vi "oa_TV Pulse Position (1Chan).vi"(4 "slope (Rising)":u16(ring) items=["Rising", "Falling"], 5 "reset? (F)":bool, 6 "pulse width (2)":i32=2, 7 "missing pulses? (no:F)":bool, 8 "error in (no error)":errorcluster, 9 "hysteresis(0)":dbl format="%.2f", 10 "threshold (auto)":dbl=inf format="%.2f", 11 "analog tacho signal":waveform(dbl)={"t0"=timestamp(0 s since 1904-01-01), "dt"=0.0, "Y"=[]}) -> (0 "error out":errorcluster, 2 "duration":dbl, 3 "pulse positions [s]":dbl[](array[numeric]))   [LabVIEW 2017, in "SoundVib_Torsional.lvlib"]
uses:
  <vilib>/addons/Sound and Vibration/Order Analysis/Torsional Vibration/SoundVib_Torsional.lvlib
  <vilib>/addons/Sound and Vibration/Order Analysis/Tach Process/SubVIs/OAT Edge Detection (1 Tach).vi
  <vilib>/addons/Sound and Vibration/Order Analysis/Tach Process/SoundVib_TachProcess.lvlib
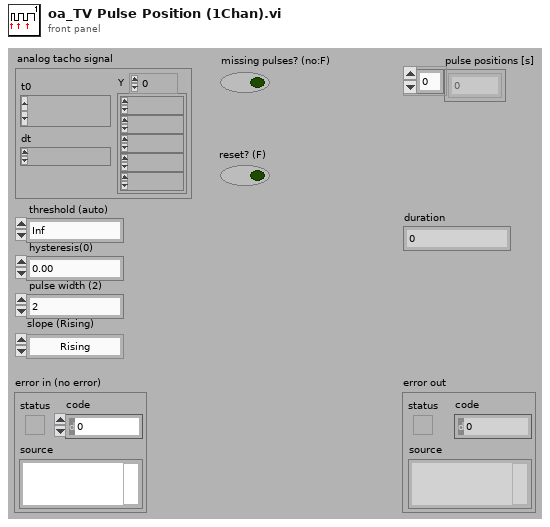
[diagram p1: front panel]
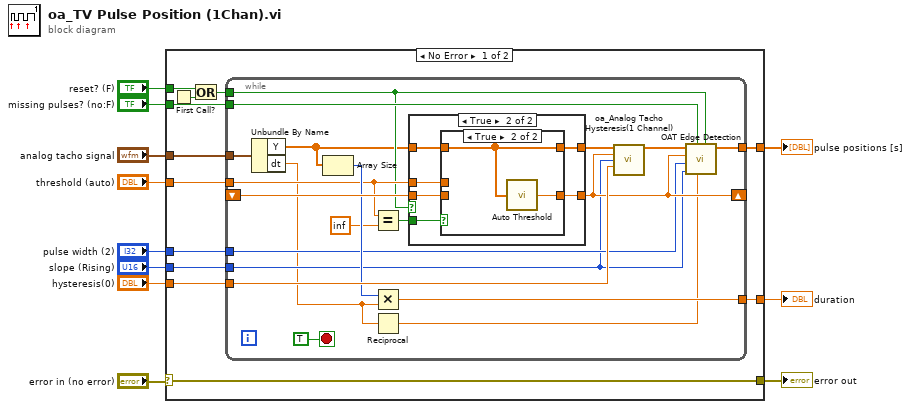
[diagram p0: block diagram]
diagram:
  n1 = case shown="No Error" "error in (no error)" {
    selector: "error in (no error)" -> [w21 w56]
    tunnel: "analog tacho signal" -> [w12 _]
    tunnel: [w21 w56] -> w10
    tunnel: "threshold (auto)" -> [w20 _]
    tunnel: [w14 _] -> w1
    tunnel: [w16 _] -> w7
    tunnel: "reset? (F)" -> [w22 _]
    tunnel: "missing pulses? (no:F)" -> [w15 _]
    tunnel: "hysteresis(0)" -> [w18 _]
    tunnel: "slope (Rising)" -> [w19 _]
    tunnel: "pulse width (2)" -> [w13 _]
    frame No Error {
      n2 = First Call?() -> (First Call?: T/F=w23:bool)
      n3 = Or(x=w22, y=w23) -> (x .or. y?=w17:bool)
      n4 = while {
        shift-right: [w33] -> _
        shift-left: _ -> [w43]
        tunnel: w17 -> [w29]
        tunnel: w20 -> [w36]
        tunnel: w19 -> [w31]
        tunnel: w18 -> [w40]
        tunnel: [w38] -> w16
        tunnel: w15 -> [w34]
        tunnel: w13 -> [w32]
        tunnel: [w27] -> w14
        tunnel: w12 -> [w24]
        stop <- TRUE stop-if-true
        n5 = Unbundle By Name(w24) -> ("Y"=w26:dbl[], "dt"=w25:dbl)
        n6 = Array Size(array=w26) -> (size(s)=w39:i32)
        n7 = Equal?(x=w36, y=inf) -> (x = y?=w35:bool)
        n8 = Multiply(x=w39, y=w25) -> (x*y=w38:dbl)
        n9 = Reciprocal(x=w25) -> (1/x=w30:dbl)
        n10 = case shown="True" w29 {
          tunnel: w26 -> [w44 w51]
          tunnel: [w45 w50] -> w33
          tunnel: w43 -> [w45 w49]
          tunnel: w36 -> [_ w48]
          tunnel: w35 -> [_ w47]
          tunnel: [w44 w46] -> w41
          frame False {
          }
          frame True {
            n11 = case shown="True" w47 {
              tunnel: w51 -> [w52 w54]
              tunnel: [w53 w55] -> w50
              tunnel: w49 -> [_ _]
              tunnel: w48 -> [w53 _]
              tunnel: [w52 w54] -> w46
              frame False {
              }
              frame True {
                n12 = call <vilib>:"Auto Threshold.vi"("x[n]"=w54) -> ("threshold"=w55:dbl)
              }
            }
          }
        }
        n13 = call <vilib>:"oa_Analog Tacho Hysteresis(1 Channel).vi"("input signal"=w41, "threshold (auto)"=w33, "slope (Rising)"=w31, "hysteresis(0)"=w40) -> ("output signal"=w28:dbl[])  [unwired: 10 in, 1 out]
        n14 = call-poly <vilib>:"OAT Edge Detection.vi"("reset? (True)"=w29, "sampling frequency [Hz]"=w30, "missing pulses? (no:F)"=w34, "slope (Rising)"=w31, "pulse width (2)"=w32, "threshold (0.0)"=w33, "x[n]"=w28) -> ("pulse positions [s]"=w27:dbl[])  [unwired: 3 in, 1 out]
      }
    }
    frame Error {
    }
  }
  "error out" <- w10
  "pulse positions [s]" <- w1
  "duration" <- w7
